vi "Refresh FPGA Bitfile Wrapper.vi"(8 "error in (no error)":errorcluster, 11 "Node Ptr":u64 format="%.0x") -> (0 "error out":errorcluster)   [LabVIEW 2015, in "Engine Simulation Toolkit System Explorer.lvlib"]
uses:
  Engine Simulation Toolkit System Explorer.lvlib
  Shared/Properties.vi
  <vilib>/NI Veristand/Custom Device API/Get Item Property (Boolean).vi
  Shared/Engine Simulation Toolkit Shared.lvlib
  <vilib>/NI VeriStand/Custom Device API/Custom Device API.lvlib
panel:
  in  "Tag":string
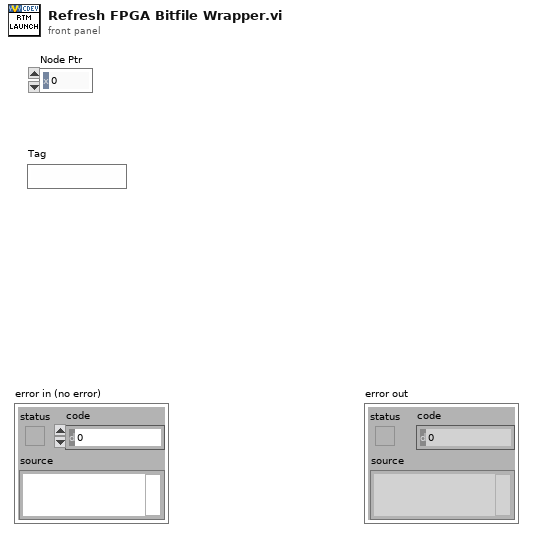
[diagram p1: front panel]
types:
  T1 = typedef "Custom Device API.lvlib/Custom Device Item Ref.ctl" = u64
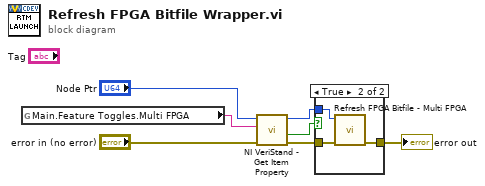
[diagram p0: block diagram]
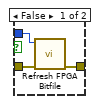
[diagram p2: hidden frame]
diagram:
  n1 = global read "Properties.vi" "Main.Feature Toggles.Multi FPGA"() -> (w1:string)
  n2 = call-poly <vilib>:"NI VeriStand - Get Item Property.vi"("error in (no error)"="error in (no error)", "Property Name"=w1, "Item Ref in"="Node Ptr") -> ("error out"=w6:errorcluster, "Value"=w5:bool, "Item Ref out"=w2:T1)  [unwired: 5 in, 1 out]
  n3 = case shown="True" w5 {
    tunnel: w6 -> [w10 w13]
    tunnel: [w9 w11] -> w7
    tunnel: w2 -> [w8 w12]
    frame False {
      n4 = call "Refresh FPGA Bitfile.vi"("error in (no error)"=w10, "Node Ptr"=w8) -> ("error out"=w9:errorcluster)  [unwired: 9 in]
    }
    frame True {
      n5 = call "Refresh FPGA Bitfile - Multi FPGA.vi"("error in (no error)"=w13, "Node Ptr"=w12) -> ("error out"=w11:errorcluster)  [unwired: 9 in]
    }
  }
  "error out" <- w7
